vi "AmbientLightSensor.vi"() -> ()   [LabVIEW 2014]
doc: "This example reads data from TEMT6000 Ambient Light sensor, processes the data and displays the data on the waveform chart."
uses:
  <vilib>/myRIO/Instrument Drivers/Onboard IO/AI/vis/Read.vi
  <vilib>/myRIO/Common/Instrument Driver Framework/myRIO v1.0/UART/vis/myRIO v1.0 Close UART.vi
  <vilib>/myRIO/Instrument Drivers/Onboard IO/AI/vis/Smart Open.vi
  <vilib>/Utility/error.llb/Error Cluster From Error Code.vi
  <vilib>/myRIO/Common/Instrument Driver Framework/myRIO v1.0/AI/vis/myRIO v1.0 Read AI.vi
  <vilib>/myRIO/Common/Instrument Driver Framework/Utilities/vis/FPGA Ref Manager.vi
  <vilib>/myRIO/Common/Instrument Driver Framework/myRIO v1.0/myRIO v1.0 Reset FPGA.vi
  <vilib>/myRIO/Common/Instrument Driver Framework/myRIO v1.0/IRQ/vis/myRIO v1.0 IRQ Info FGV.vi
  <vilib>/myRIO/Common/Instrument Driver Framework/myRIO v1.0/IRQ/vis/myRIO v1.0 Timer IRQ Info FGV.vi
  <vilib>/myRIO/Common/Instrument Driver Framework/myRIO v1.0/IRQ/vis/myRIO v1.0 ISR Agent.vi
  <vilib>/myRIO/Instrument Drivers/Utilities/Utilities.lvlib
panel:
  out "error out":errorcluster
  in  "Stop":bool
  out "Light Waveform":dbl(graph)
  # "Overview: This example reads data from TEMT6000 Ambient Light sensor, processes the data and displays the data on the waveform chart.\nRequirements: LabVIEW Full Development System\nInstructions:\n1. Connect the sensor to myRIO.\n     TEMT 6000                             myRIO\n      VCC                                         +5V\n      Gnd                                         Gnd\n      SIG                                           Connector A/AI0\n2. Check the myRIO target IP Address in the project and make sure the target IP Address is correct.\n3. Run this VI."
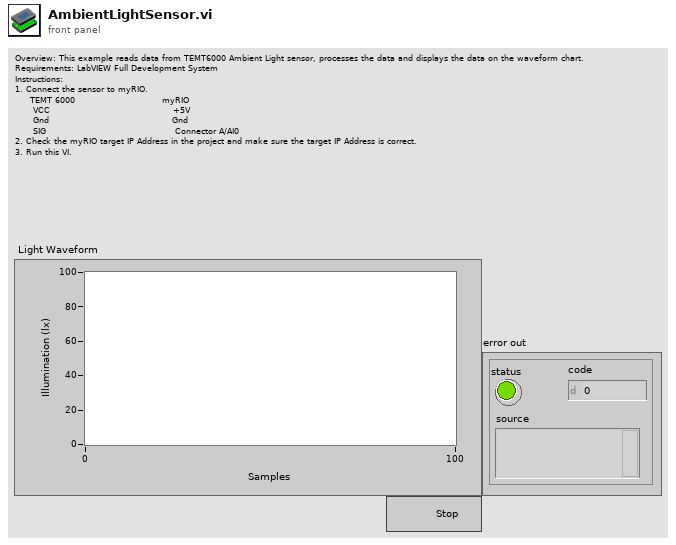
[diagram p1: front panel]
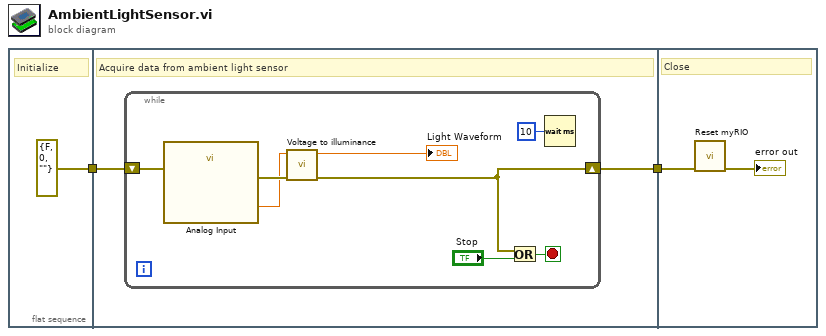
[diagram p0: block diagram]
diagram:
  n1 = flat-sequence {
    tunnel: [errorcluster {"status"=FALSE, "code"=0, "source"=""} ("error out")] -> w1
    tunnel: [w5] -> w2
    tunnel: w1 -> [w4]
    tunnel: w2 -> [w15]
    frame #0 {
      # "Initialize"
    }
    frame #1 {
      # "Acquire data from ambient light sensor"
      n2 = while {
        shift-right: [w8] -> w5
        shift-left: w4 -> [w10]
        stop <- w12 stop-if-true
        n3 = call "Analog Input"("error in (no error)"=w10) -> ("A/AI0 (Pin 3)"=w6:dbl, "error out"=w9:errorcluster)  [unwired: 25 in]
        n4 = call "Voltage to illuminance.vi"("error in (no error)"=w9, "Input Voltage (V)"=w6) -> ("error out"=w8:errorcluster, "Illuminance (lx)"=→"Light Waveform":dbl)  [unwired: 8 in]
        n5 = Or(x=w8, y="Stop") -> (x .or. y?=w12:bool)
        n6 = Wait (ms)(milliseconds to wait=u32 10) -> ()  [unwired: 1 out]
      }
    }
    frame #2 {
      # "Close"
      n7 = call <vilib>:"Reset myRIO.vi"("error in (no error)"=w15) -> ("error out"=→"error out":errorcluster)  [unwired: 10 in]
    }
  }
